vi "Test Internal Logic.vi"() -> ()   [LabVIEW 2020, in "Tamer.lvlib" / "Tamer.lvclass"]
uses:
  Tamer.lvclass
  Run Utilities/TypeDefs/Synchronize FPGA Cluster.ctl
  <vilib>/Utility/miscctls.llb/LVComboBoxStrsAndValuesArrayTypeDef.ctl
  Monkey Summary.ctl
  Run Utilities/TypeDefs/Monkey Status.ctl
  Link Chain GUI.ctl
  Reply.ctl
  Run Utilities/TypeDefs/Messages/Script Checker Message.ctl
  Run Utilities/TypeDefs/Script Checker Result.ctl
  af21684e-d11e-44f0-8b97-6f30b353b7a1.vi
  <vilib>/numeric/Random Number (Range) U64.vi
  d09a2809-11e4-490a-8cc9-e655e83ef35e.vi
  8c686b44-d516-4979-b4c0-187cf11809c2.vi
  <vilib>/numeric/sub_Random U32.vi
  <vilib>/Comparison/Less/Less Functor/Less Functor.lvclass
  Run Utilities/Run Utilities.lvlib
panel:
  in  "stop":bool
  in  "Tab Control":T1(tab)
  in  "Sync. Mask":T2[](array[typedef])=[{"Status"=FALSE, "FPGA Name"="Kasli 1"}, {"Status"=FALSE, "FPGA Name"="Kasli 1"}, {"Status"=TRUE, "FPGA Name"="Kasli 1"}]
  out "Synced Kaslis":string[](array[string])
  out "Number of Kaslis":i32
  out "Sync Process ID":string
  out "Processes":map{string, string[]}(c390)
  out "Synced Monkeys":string[](array[string])
  out "Number of Monkeys":i32
  out "key not found?":bool
  in  "Return Code recieved":string
  out "Return Code de-coded":T3(ring)
  in  "Status":string
  out "Status (enum)":T4=enum."Ongoing"
  in  "1D array in":string[](array[string])=["a00", "a01", "a10", "a11", "a20", "a21"]
  in  "columns":u32=1 min=1
  out "1D to 2D arry out":string[][](array[string])
  out "2D to 1D array out":string[](array[string])
  out "output array":T5
  in  "ADD":bool
  in  "REMOVE":bool
  in  "RESET":bool
  out "Value":string
  in  "Proc. Selector":string(combo)
  out "Size":i32
  out "added/deleted portion":cluster{"String":string, "Value":string}
  out "selected item":cluster{"String":string, "Value":string}
  in  "new Monkey":T6={"Color"=16777238, "Status"=enum."Init", "Continuous"=FALSE, "Scripts left"=0, "Scripts skipped"=0, "ETA"="", "Current Action"="", "Report from previous RUNs"="", "Monkey ID"="", "With DAQ?"=FALSE, "Linked?"=FALSE, "Paused"=FALSE}
  in  "Index":i32
  in  "SPAWN":bool
  in  "KILL":bool
  in  "KILL ALL":bool
  out "The Stage":T6[][](array[typedef])
  out "Monkey ID selected":string
  out "Guardians that have replied (unsorted)":T8[](array[typedef])
  out "Guardians that have replied (sorted)":T8[](array[typedef])
  out "Script Checker Results (unsorted)":T9[](array[typedef])
  out "Script Checker Results (sorted)":T9[](array[typedef])
  in  "Sync. Mask":T2[](array[typedef])=[{"Status"=FALSE, "FPGA Name"="Kasli 1"}, {"Status"=FALSE, "FPGA Name"="Kasli 1"}, {"Status"=TRUE, "FPGA Name"="Kasli 1"}]
  out "Kaslis":map{string, string}(c390)
  out "Monkeys Status in":map{string, T4}(c390)
  out "Monkeys":map{string, string[]}(c390)
  out "Processes in":map{string, string[]}(c390)
  out "Monkeys Status out":map{string, T4}(c390)
  out "Processes out":map{string, string[]}(c390)
  out "Kaslis out":map{string, string}(c390)
  out "Monkeys out":map{string, string[]}(c390)
  out "Sync Process ID":string
  in  "Monkey ID":string
  out "Sync Mask out":T2[](array[typedef])
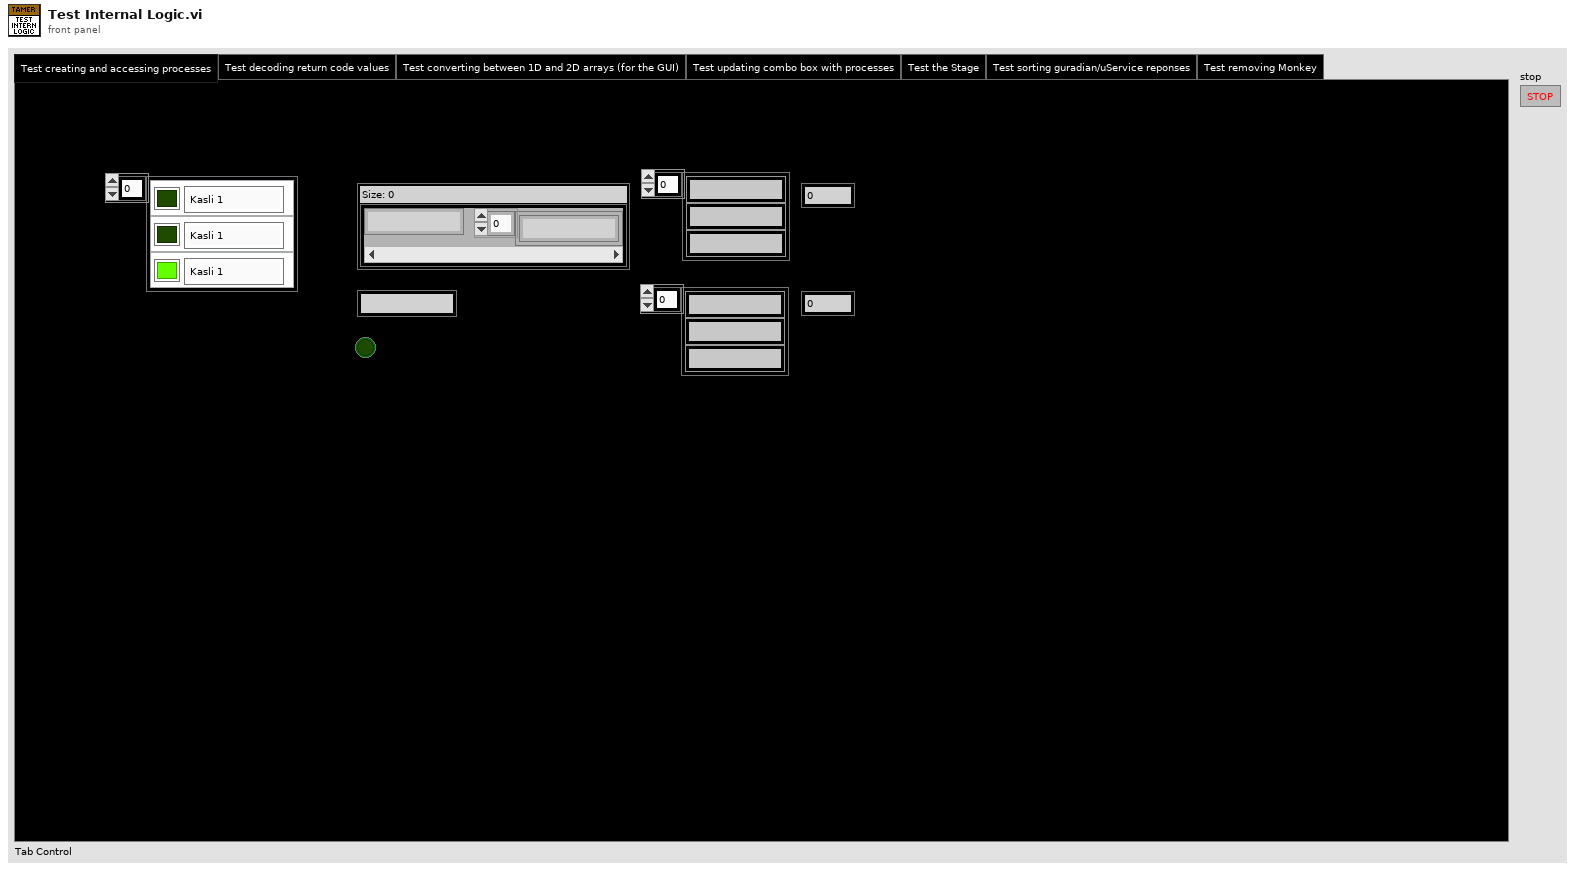
[diagram p1: front panel]
types:
  T1 = enum32{"Test creating and accessing processes", "Test decoding return code values", "Test converting between 1D and 2D arrays (for the GUI)", "Test updating combo box with processes", "Test the Stage", "Test sorting guradian/uService reponses", "Test removing Monkey"}
  T2 = typedef "Run Utilities.lvlib/Synchronize FPGA Cluster.ctl" = cluster{"Status":bool, "FPGA Name":string}
  T3 = enum16{"All Good", "Retry", "Skip", "Skip All", "ABORT"}
  T4 = typedef "Run Utilities.lvlib/Monkey Status.ctl" = enum16{"Init", "Paused", "Ongoing", "Stopped", "Finished (no errors)", "Finished (with errors)"}
  T5 = typedef "LVComboBoxStrsAndValuesArrayTypeDef.ctl" = cluster{"String":string, "Value":string}[]
  T6 = typedef "Tamer.lvlib/Tamer.lvclass/Monkey Summary.ctl" = cluster{"Color":u32, "Status":T4, "Continuous":bool, "Scripts left":u32, "Scripts skipped":u32, "ETA":string, "Current Action":string, "Report from previous RUNs":string, "Monkey ID":string, "With DAQ?":bool, "Linked?":T7, "Paused":bool}
  T7 = typedef "Tamer.lvlib/Tamer.lvclass/Link Chain GUI.ctl" = bool
  T8 = typedef "Tamer.lvlib/Tamer.lvclass/Reply.ctl" = cluster{"ID":string, "Status":bool, "GUID":string}
  T9 = typedef "Run Utilities.lvlib/Script Checker Message.ctl" = cluster{"Monkey ID":string, "Script Checker Result":T10}
  T10 = typedef "Run Utilities.lvlib/Script Checker Result.ctl" = enum16{"Passed", "Failed", "Empty"}
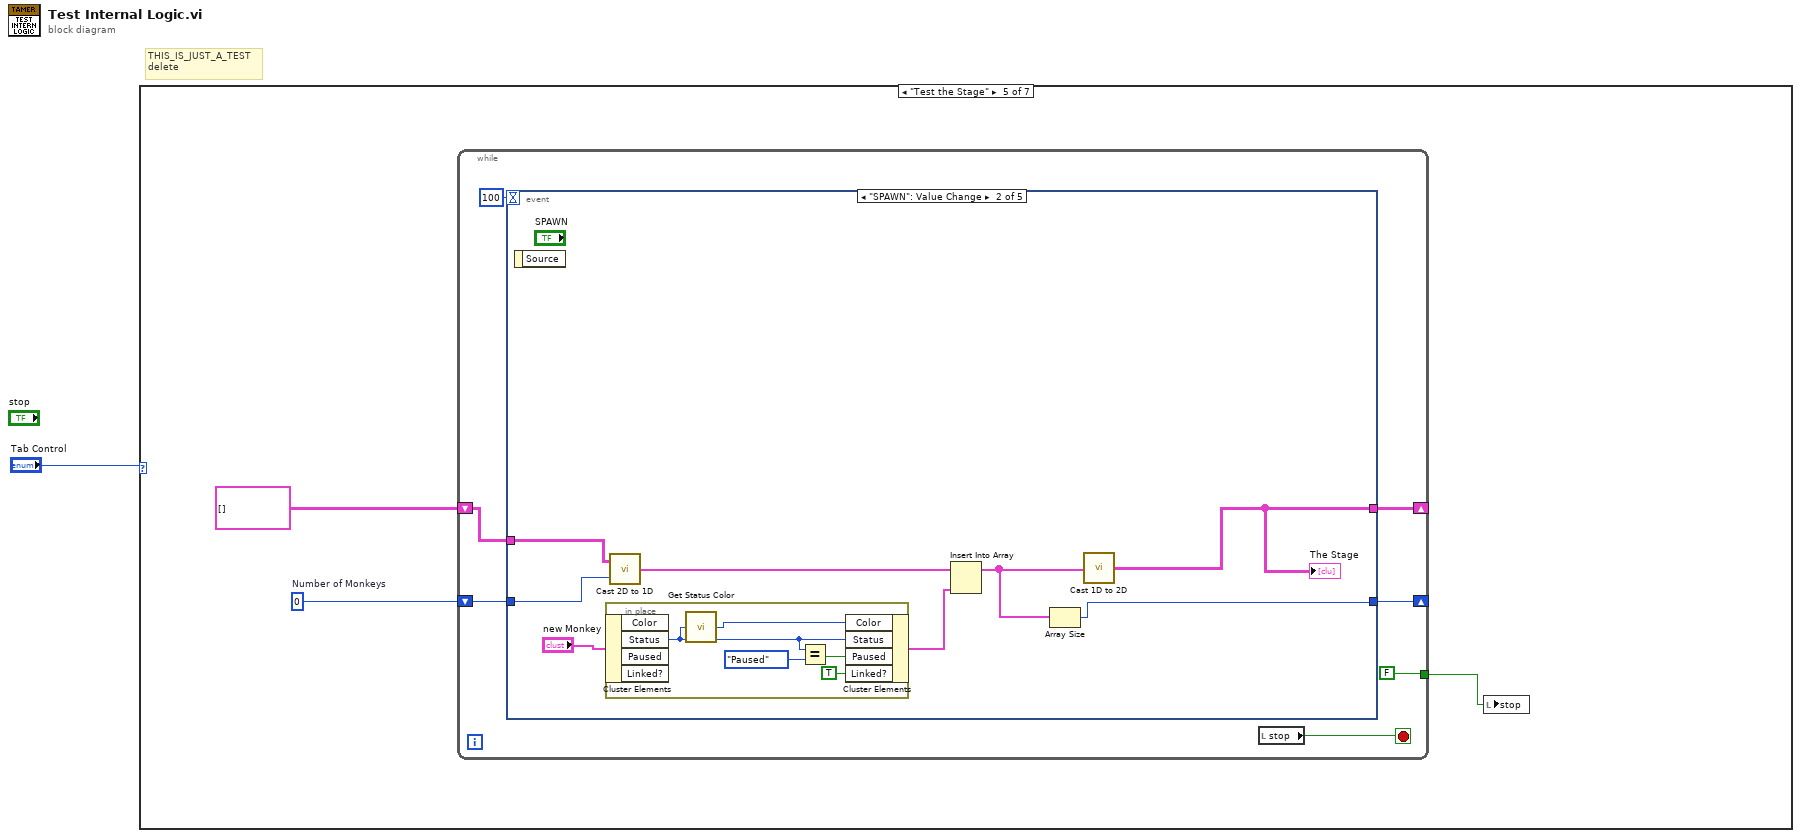
[diagram p0: block diagram]
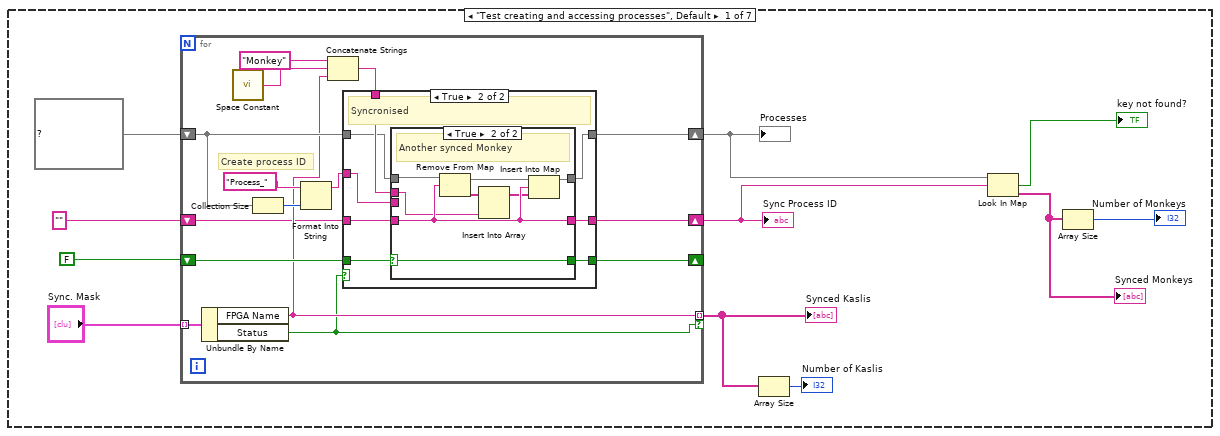
[diagram p2: hidden frame]
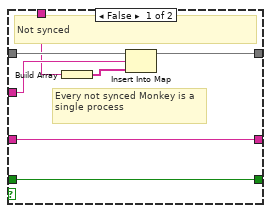
[diagram p3: hidden frame]
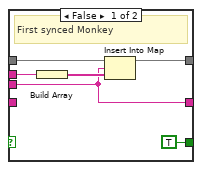
[diagram p4: hidden frame]
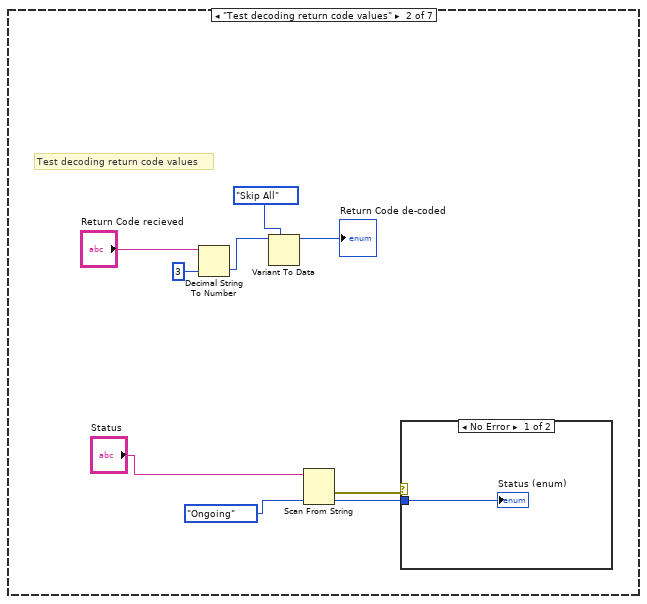
[diagram p5: hidden frame]
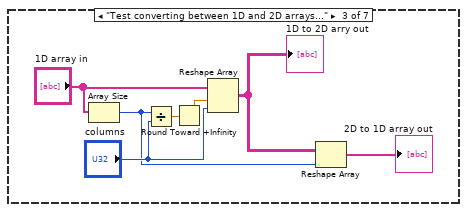
[diagram p7: hidden frame]
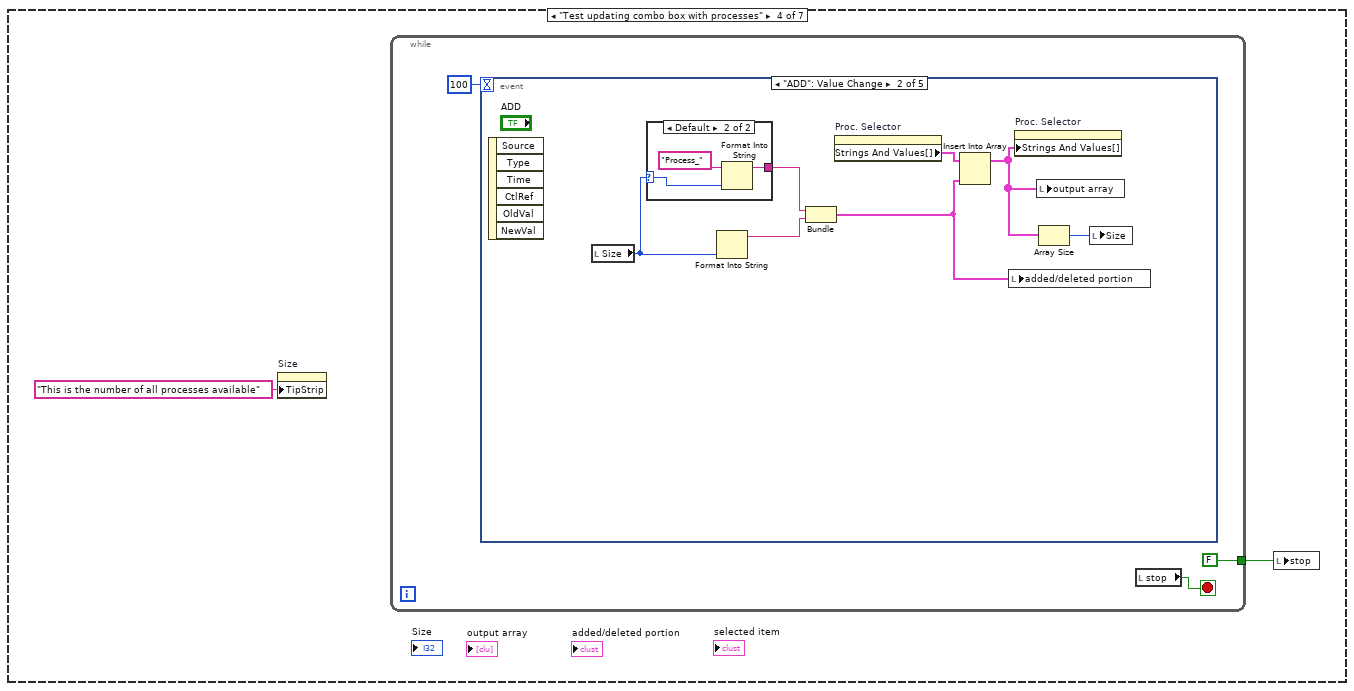
[diagram p8: hidden frame]
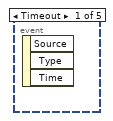
[diagram p9: hidden frame]
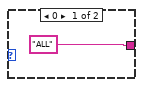
[diagram p10: hidden frame]
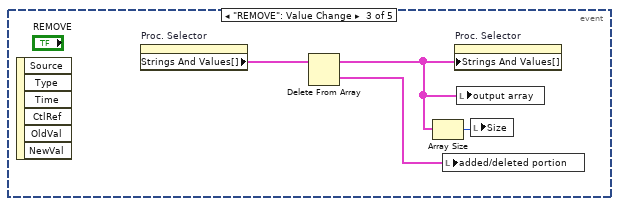
[diagram p11: hidden frame]
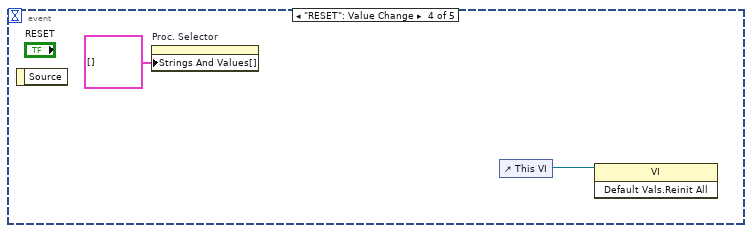
[diagram p12: hidden frame]
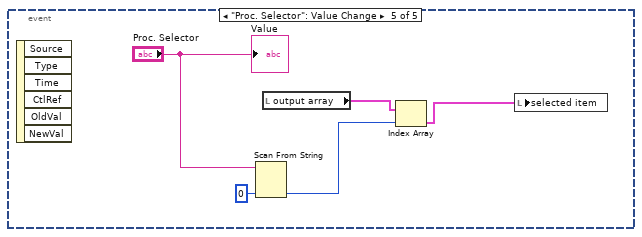
[diagram p13: hidden frame]
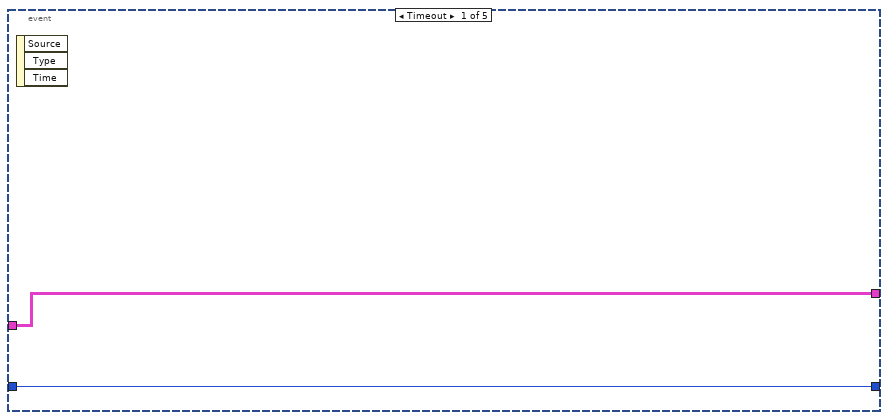
[diagram p14: hidden frame]
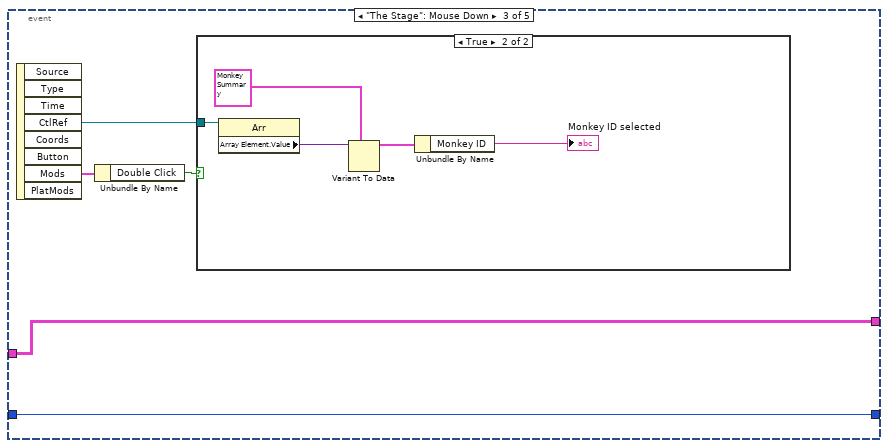
[diagram p15: hidden frame]
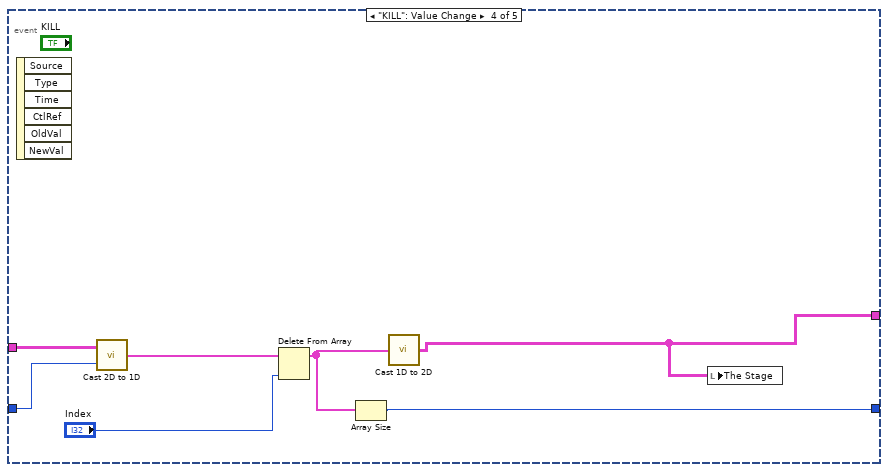
[diagram p17: hidden frame]
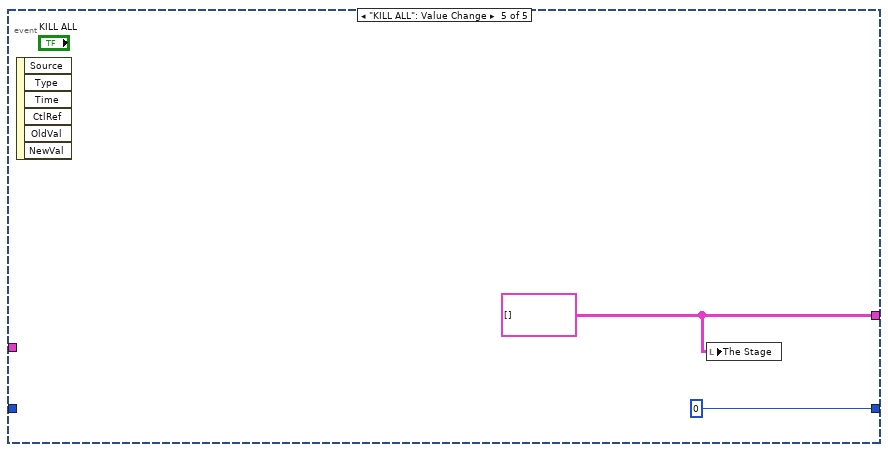
[diagram p18: hidden frame]
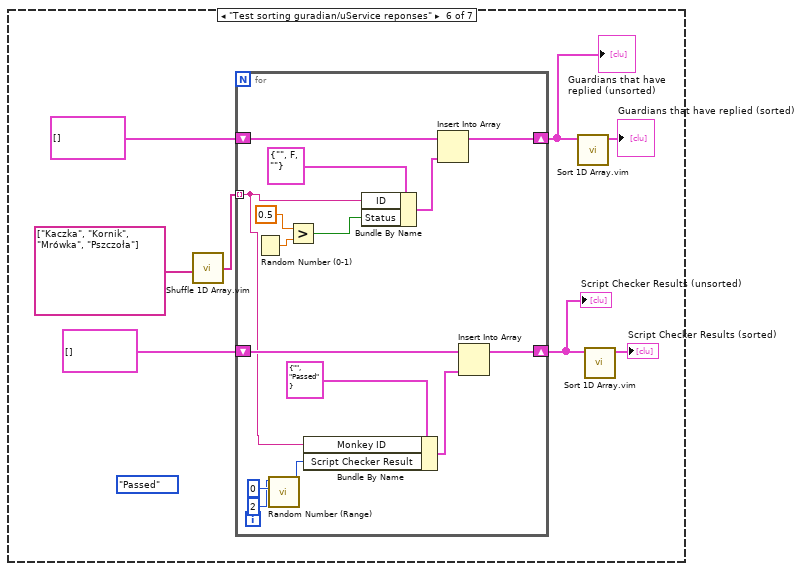
[diagram p19: hidden frame]
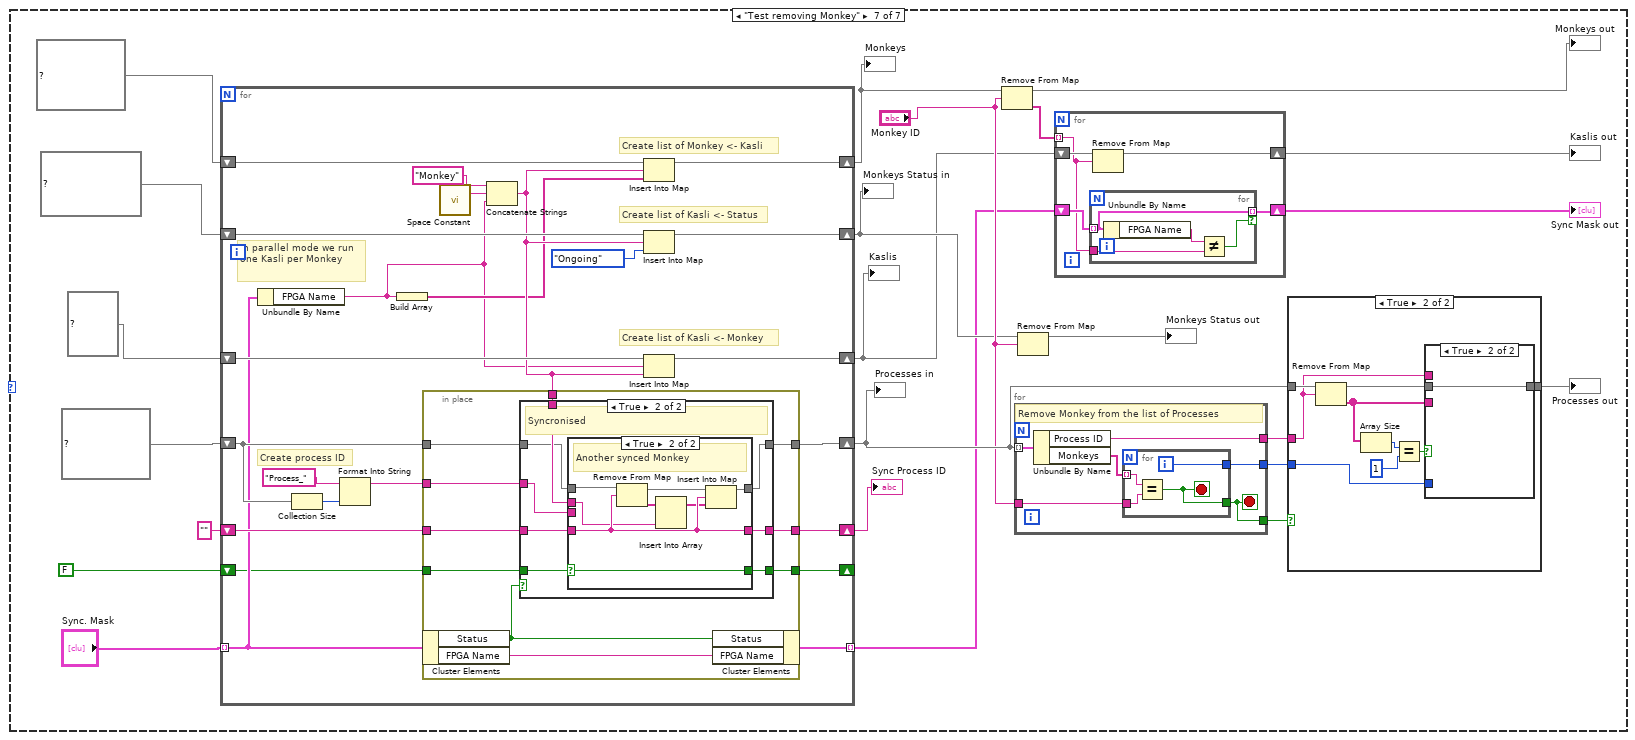
[diagram p20: hidden frame]
diagram:
  # "THIS_IS_JUST_A_TEST\ndelete"
  n1 = case shown="\"Test the Stage\"" "Tab Control" {
    frame "Test creating and accessing processes", Default {
      n2 = for {
        tunnel: "Sync. Mask" -> [w27] mode=indexing
        tunnel: [w17] -> w3 mode=indexing if=w13
        shift-right: [w26] -> w8
        shift-left: map{string, string[]} {} ("Processes") -> [w23]
        shift-right: [w21] -> _
        shift-left: FALSE ("Sync. Process added") -> [w22]
        shift-right: [w15] -> w9
        shift-left: "" -> [w14]
        # "Create process ID"
        n3 = Unbundle By Name(w27) -> ("FPGA Name"=w17:string, "Status"=w13:bool)
        n4 = call <vilib>:"Space Constant.vi"() -> ("String"=w18:string)
        n5 = Collection Size(1:w23) -> (0:w25:i32)
        n6 = Format Into String(initial string="Process_", w25) -> (resulting string=w20:string)  [unwired: 2 in, 1 out]
        n7 = Concatenate Strings("Monkey" ("string"), w18, w17) -> (w16:string)
        n8 = case shown="True" w13 {
          tunnel: w20 -> [w32 w38]
          tunnel: w23 -> [w34 w39]
          tunnel: [w33 w37] -> w26
          tunnel: w16 -> [w30 w41]
          tunnel: w22 -> [w29 w42]
          tunnel: [w29 w40] -> w21
          tunnel: [w28 w36] -> w15
          tunnel: w14 -> [w28 w35]
          frame False {
            # "Every not synced Monkey is a single process"
            # "Not synced"
            n9 = Build Array(w30) -> (w31:string[])
            n10 = Insert Into Map(map in=w34, key=w32, value=w31) -> (map out=w33:map{string, string[]})  [unwired: 2 out]
          }
          frame True {
            # "Syncronised"
            n11 = case shown="True" w42 {
              selector: w42 -> [_ w56]
              tunnel: [w46 w54] -> w37
              tunnel: w39 -> [w47 w55]
              tunnel: w41 -> [w45 w50]
              tunnel: [TRUE w56] -> w40
              tunnel: w38 -> [w43 _]
              tunnel: [w43 w52] -> w36
              tunnel: w35 -> [_ w52]
              frame False {
                # "First synced Monkey"
                n12 = Build Array(w45) -> (w44:string[])
                n13 = Insert Into Map(map in=w47, key=w43, value=w44) -> (map out=w46:map{string, string[]})  [unwired: 2 out]
              }
              frame True {
                # "Another synced Monkey"
                n14 = Remove From Map(10:w52, 11:w55) -> (1:w51:string[], 3:w53:map{string, string[]})  [unwired: 1 out]
                n15 = Insert Into Array(array=w51, new element=w50) -> (w49:string[])  [unwired: 1 in]
                n16 = Insert Into Map(map in=w53, key=w52, value=w49) -> (map out=w54:map{string, string[]})  [unwired: 2 out]
              }
            }
          }
        }
      }
      "Synced Kaslis" <- w3
      "Sync Process ID" <- w9
      "Processes" <- w8
      n17 = Array Size(array=w3) -> (size(s)=→"Number of Kaslis":i32)
      n18 = Look In Map(map=w8, key=w9) -> (key not found?=→"key not found?":bool, value=w10:string[])  [unwired: 1 in]
      "Synced Monkeys" <- w10
      n19 = Array Size(array=w10) -> (size(s)=→"Number of Monkeys":i32)
    }
    frame "Test decoding return code values" {
      # "Test decoding return code values"
      n20 = Decimal String To Number(string="Return Code recieved", default (0L)=3) -> (number=w65:i32)  [unwired: 1 in, 1 out]
      n21 = Variant To Data(type=T3."Skip All" ("Return Code"), Variant=w65) -> (data=→"Return Code de-coded":T3)  [unwired: 1 in, 1 out]
      n22 = Scan From String(input string="Status", default 1=Monkey_Status."Ongoing" ("Monkey Status")) -> (error out=w57:errorcluster, output 1=w58:T4)  [unwired: 3 in, 2 out]
      n23 = case shown="No Error" w57 {
        tunnel: w58 -> [w66 _]
        frame No Error {
          "Status (enum)" <- w66
        }
        frame Error {
        }
      }
    }
    frame "Test converting between 1D and 2D arrays (for the GUI)" {
      n24 = Array Size(array="1D array in") -> (size(s)=w69:i32)
      n25 = Divide(x=w69, y="columns") -> (x/y=w68:dbl)
      n26 = Round Toward +Infinity(x=w68) -> (ceil(x): smallest int >= x=w67:dbl)
      n27 = Reshape Array("1D array in", w67, "columns") -> (w71:string[][])
      "1D to 2D arry out" <- w71
      n28 = Reshape Array(w71, w69) -> (→"2D to 1D array out":string[])
    }
    frame "Test updating combo box with processes" {
      n29 = property on="Size" class="DigNum (strict)"("TipStrip"="This is the number of all processes available" ("Tip Strip")) -> ()  [unwired: 2 in, 2 out]
      n30 = while {
        tunnel: [FALSE] -> w75
        stop <- w77 stop-if-true
        n31 = event shown="[1] \"ADD\": Value Change" {
          selector: _ -> [_ _ _ _ _]
          dyn-events: _ -> [_ _ _ _ _]
          timeout: 100 -> [_ _ _ _ _]
          event Timeout {
            n32 = event-data() -> ()  [unwired: 1 in, 3 out]
          }
          event "ADD": Value Change {
            n33 = event-data() -> ()  [unwired: 1 in, 6 out]
            n34 = local read "Size"() -> (w82:i32)
            n35 = case shown="Default" w82 {
              selector: w82 -> [_ w88]
              tunnel: ["ALL" w87] -> w84
              frame 0 {
              }
              frame Default {
                n36 = Format Into String(initial string="Process_" ("string"), w88) -> (resulting string=w87:string)  [unwired: 2 in, 1 out]
              }
            }
            n37 = Format Into String(w82) -> (resulting string=w83:string)  [unwired: 3 in, 1 out]
            n38 = Bundle(w84, w83) -> (w79:cluster{string, string})  [unwired: 1 in]
            n39 = property on="Proc. Selector" class="CmbBox"() -> ("Strings And Values[]"=w85:T5)  [unwired: 2 in, 2 out]
            n40 = Insert Into Array(array=w85, new element=w79) -> (w80:T5)  [unwired: 1 in]
            n41 = local write "added/deleted portion"(w79) -> ()
            n42 = property on="Proc. Selector" class="CmbBox"("Strings And Values[]"=w80) -> ()  [unwired: 2 in, 2 out]
            n43 = local write "output array"(w80) -> ()
            n44 = Array Size(array=w80) -> (size(s)=w81:i32)
            n45 = local write "Size"(w81) -> ()
          }
          event "REMOVE": Value Change {
            n46 = event-data() -> ()  [unwired: 1 in, 6 out]
            n47 = property on="Proc. Selector" class="CmbBox"() -> ("Strings And Values[]"=w93:T5)  [unwired: 2 in, 2 out]
            n48 = Delete From Array(array=w93) -> (deleted portion=w92:cluster{"String":string, "Value":string}, array with subset deleted=w90:T5)  [unwired: 2 in]
            n49 = Array Size(array=w90) -> (size(s)=w91:i32)
            n50 = local write "added/deleted portion"(w92) -> ()
            n51 = property on="Proc. Selector" class="CmbBox"("Strings And Values[]"=w90) -> ()  [unwired: 2 in, 2 out]
            n52 = local write "output array"(w90) -> ()
            n53 = local write "Size"(w91) -> ()
          }
          event "RESET": Value Change {
            n54 = event-data() -> ()  [unwired: 1 in, 1 out]
            n55 = property on="Proc. Selector" class="CmbBox"("Strings And Values[]"=T5 [] ("Strings And Values []")) -> ()  [unwired: 2 in, 2 out]
            n56 = control-ref of="This VI"() -> (w95:refnum<vi>)
            n57 = invoke class="VI" method="Default Vals.Reinit All"(reference=w95) -> ()  [unwired: 2 in, 3 out]
          }
          event "Proc. Selector": Value Change {
            n58 = event-data() -> ()  [unwired: 1 in, 6 out]
            n59 = Scan From String(input string="Proc. Selector", default 1=0) -> (output 1=w96:i32)  [unwired: 3 in, 3 out]
            n60 = local read "output array"() -> (w100:T5)
            n61 = Index Array(array=w100, index=w96) -> (element=w99:cluster{"String":string, "Value":string})
            n62 = local write "selected item"(w99) -> ()
            "Value" <- "Proc. Selector"
          }
        }
        n63 = local read "stop"() -> (w77:bool)
      }
      n64 = local write "stop"(w75) -> ()
    }
    frame "Test the Stage" {
      w102 = 0  # Number of Monkeys
      n65 = while {
        shift-right: [w108] -> _
        shift-left: w102 -> [w109]
        shift-right: [w105] -> _
        shift-left: T6[][] [] ("The Cage") -> [w104]
        tunnel: [FALSE] -> w103
        stop <- w107 stop-if-true
        n66 = event shown="[1] \"SPAWN\": Value Change" {
          selector: _ -> [_ _ _ _ _]
          dyn-events: _ -> [_ _ _ _ _]
          timeout: 100 -> [_ _ _ _ _]
          tunnel: w109 -> [w112 w115 w128 w137 _]
          tunnel: [w111 w119 w129 w141 w143] -> w105
          tunnel: [w112 w117 w128 w139 0 ("Number of Monkeys")] -> w108
          tunnel: w104 -> [w111 w116 w129 w138 _]
          event Timeout {
            n67 = event-data() -> ()  [unwired: 1 in, 3 out]
          }
          event "SPAWN": Value Change {
            n68 = event-data() -> ()  [unwired: 1 in, 1 out]
            n69 = in-place {
              n70 = in-place-cluster #1("new Monkey") -> ("Status"=w124:T4)  [unwired: 3 out]
              n71 = call "Get Status Color.vi"("Monkey Status"=w124) -> ("Color"=w125:u32)
              n72 = Equal?(x=w124, y=Monkey_Status."Paused") -> (x = y?=w122:bool)
              n73 = in-place-cluster #1("Color"=w125, "Status"=w124, "Paused"=w122, "Linked?"=T7 TRUE) -> (w120:T6)
            }
            n74 = call "Cast 2D to 1D.vi"("1D size"=w115, "2D Synchronous Monkeys"=w116) -> ("1D Synchronous Monkeys"=w114:T6[])
            n75 = Insert Into Array(array=w114, new element=w120) -> (w118:T6[])  [unwired: 1 in]
            n76 = Array Size(array=w118) -> (size(s)=w117:i32)
            n77 = call "Cast 1D to 2D.vi"("1D Monkeys"=w118) -> ("2D Monkeys"=w119:T6[][])
            "The Stage" <- w119
          }
          event "The Stage": Mouse Down {
            n78 = event-data() -> ("CtlRef"=w130:refnum<vi>, "Mods"=w127:cluster{"Double Click":bool, "Menu Key":bool})  [unwired: 1 in, 6 out]
            n79 = Unbundle By Name(w127) -> ("Double Click"=w126:bool)
            n80 = case shown="True" w126 {
              tunnel: w130 -> [_ w135]
              frame False {
              }
              frame True {
                n81 = property class="Arr"(reference=w135) -> ("Array Element.Value"=w134:variant)  [unwired: 1 in, 2 out]
                n82 = Variant To Data(type=T6 {"Color"=16777238, "Status"=enum."Init", "Continuous"=FALSE, "Scripts left"=0, "Scripts skipped"=0, "ETA"="", "Current Action"="", "Report from previous RUNs"="", "Monkey ID"="", "With DAQ?"=FALSE, "Linked?"=FALSE, "Paused"=FALSE} ("Monkey Summary"), Variant=w134) -> (data=w133:T6)  [unwired: 1 in, 1 out]
                n83 = Unbundle By Name(w133) -> ("Monkey ID"=→"Monkey ID selected":string)
              }
            }
          }
          event "KILL": Value Change {
            n84 = event-data() -> ()  [unwired: 1 in, 6 out]
            n85 = call "Cast 2D to 1D.vi"("1D size"=w137, "2D Synchronous Monkeys"=w138) -> ("1D Synchronous Monkeys"=w136:T6[])
            n86 = Delete From Array(array=w136, index="Index") -> (array with subset deleted=w140:T6[])  [unwired: 1 in, 1 out]
            n87 = Array Size(array=w140) -> (size(s)=w139:i32)
            n88 = call "Cast 1D to 2D.vi"("1D Monkeys"=w140) -> ("2D Monkeys"=w141:T6[][])
            n89 = local write "The Stage"(w141) -> ()
          }
          event "KILL ALL": Value Change {
            w143 = T6[][] [] ("The Cage")
            n90 = event-data() -> ()  [unwired: 1 in, 6 out]
            n91 = local write "The Stage"(w143) -> ()
          }
        }
        n92 = local read "stop"() -> (w107:bool)
      }
      n93 = local write "stop"(w103) -> ()
    }
    frame "Test sorting guradian/uService reponses" {
      (unwired) Script_Checker_Result."Passed" ("Script Checker Result")
      n94 = call "Shuffle 1D Array.vim"("array"=string[] ["Kaczka", "Kornik", "Mrówka", "Pszczoła"]) -> ("shuffled array"=w151:string[])  [unwired: 4 in]
      n95 = for {
        shift-right: [w166] -> w149
        shift-left: T8[] [] ("Guardians that have replied") -> [w167]
        tunnel: w151 -> [w157] mode=indexing
        shift-right: [w159] -> w145
        shift-left: T9[] [] -> [w160]
        n96 = Random Number (0-1)() -> (number: 0 to 1=w163:dbl)
        n97 = call-poly <vilib>:"Random Number (Range).vi"("lower bound (0)"=u64 0, "upper bound (100)"=u64 2) -> ("number"=w154:u64)  [unwired: 9 in]
        n98 = Greater?(x=0.5, y=w163) -> (0:w161:bool)
        n99 = Bundle By Name(cluster=T9 {"Monkey ID"="", "Script Checker Result"=enum."Passed"} ("Message"), "Monkey ID"=w157, "Script Checker Result"=w154) -> (w153:T9)
        n100 = Bundle By Name(cluster=T8 {"ID"="", "Status"=FALSE, "GUID"=""} ("new element/subarray"), "ID"=w157, "Status"=w161) -> (w164:T8)
        n101 = Insert Into Array(array=w167, new element=w164) -> (w166:T8[])  [unwired: 1 in]
        n102 = Insert Into Array(array=w160, new element=w153) -> (w159:T9[])  [unwired: 1 in]
      }
      "Guardians that have replied (unsorted)" <- w149
      "Script Checker Results (unsorted)" <- w145
      n103 = call "Sort 1D Array.vim"("unsorted array"=w149) -> ("sorted array"=→"Guardians that have replied (sorted)":T8[])  [unwired: 10 in]
      n104 = call "Sort 1D Array.vim"("unsorted array"=w145) -> ("sorted array"=→"Script Checker Results (sorted)":T9[])  [unwired: 10 in]
    }
    frame "Test removing Monkey" {
      n105 = for {
        shift-right: [w248] -> w182
        shift-left: map{string, string[]} {} ("Monkeys") -> [w249]
        shift-right: [w246] -> w172
        shift-left: map{string, string} {} ("Kaslis") -> [w247]
        shift-right: [w244] -> w175
        shift-left: map{string, T4} {} ("Monkeys Status") -> [w245]
        tunnel: "Sync. Mask" -> [w234] mode=indexing
        tunnel: [w243] -> w169 mode=indexing
        shift-right: [w242] -> w180
        shift-left: map{string, string[]} {} ("Processes") -> [w239]
        shift-right: [w241] -> _
        shift-left: FALSE ("Sync. Process added") -> [w233]
        shift-right: [w235] -> w183
        shift-left: "" -> [w237]
        # "Create list of Kasli <- Monkey"
        # "Create list of Kasli <- Status"
        # "Create list of Monkey <- Kasli"
        # "Create process ID"
        # "In parallel mode we run one Kasli per Monkey"
        n106 = Unbundle By Name(w234) -> ("FPGA Name"=w227:string)
        n107 = Collection Size(1:w239) -> (0:w240:i32)
        n108 = Format Into String(initial string="Process_", w240) -> (resulting string=w236:string)  [unwired: 2 in, 1 out]
        n109 = Build Array(w227) -> (w228:string[])
        n110 = call <vilib>:"Space Constant.vi"() -> ("String"=w231:string)
        n111 = Concatenate Strings("Monkey" ("string"), w231, w227) -> (w229:string)
        n112 = in-place {
          in-place-border: [w256] -> w242
          in-place-border: w239 -> [w257]
          in-place-border: w233 -> [w253]
          in-place-border: [w252] -> w241
          in-place-border: w236 -> [w258]
          in-place-border: w229 -> [w255]
          in-place-border: w237 -> [w254]
          in-place-border: [w251] -> w235
          n113 = in-place-cluster #2(w234) -> ("Status"=w250:bool, "FPGA Name"=w259:string)
          n114 = case shown="True" w250 {
            tunnel: w258 -> [w264 w270]
            tunnel: w257 -> [w266 w271]
            tunnel: [w265 w269] -> w256
            tunnel: w255 -> [w262 w273]
            tunnel: w254 -> [w261 w267]
            tunnel: w253 -> [w260 w274]
            tunnel: [w260 w272] -> w252
            tunnel: [w261 w268] -> w251
            frame False {
              # "Every not synced Monkey is a single process"
              # "Not synced"
              n115 = Build Array(w262) -> (w263:string[])
              n116 = Insert Into Map(map in=w266, key=w264, value=w263) -> (map out=w265:map{string, string[]})  [unwired: 2 out]
            }
            frame True {
              # "Syncronised"
              n117 = case shown="True" w274 {
                selector: w274 -> [_ w288]
                tunnel: [w278 w286] -> w269
                tunnel: w271 -> [w279 w287]
                tunnel: w273 -> [w277 w282]
                tunnel: [TRUE w288] -> w272
                tunnel: w270 -> [w275 _]
                tunnel: [w275 w284] -> w268
                tunnel: w267 -> [_ w284]
                frame False {
                  # "First synced Monkey"
                  n118 = Build Array(w277) -> (w276:string[])
                  n119 = Insert Into Map(map in=w279, key=w275, value=w276) -> (map out=w278:map{string, string[]})  [unwired: 2 out]
                }
                frame True {
                  # "Another synced Monkey"
                  n120 = Remove From Map(10:w284, 11:w287) -> (1:w283:string[], 3:w285:map{string, string[]})  [unwired: 1 out]
                  n121 = Insert Into Array(array=w283, new element=w282) -> (w281:string[])  [unwired: 1 in]
                  n122 = Insert Into Map(map in=w285, key=w284, value=w281) -> (map out=w286:map{string, string[]})  [unwired: 2 out]
                }
              }
            }
          }
          n123 = in-place-cluster #2("Status"=w250, "FPGA Name"=w259) -> (w243:T2)
        }
        n124 = Insert Into Map(map in=w249, key=w229, value=w228) -> (map out=w248:map{string, string[]})  [unwired: 2 out]
        n125 = Insert Into Map(map in=w245, key=w229, value=Monkey_Status."Ongoing") -> (map out=w244:map{string, T4})  [unwired: 2 out]
        n126 = Insert Into Map(map in=w247, key=w227, value=w229) -> (map out=w246:map{string, string})  [unwired: 2 out]
      }
      "Kaslis" <- w172
      "Monkeys" <- w182
      "Monkeys Status in" <- w175
      "Processes in" <- w180
      "Sync Process ID" <- w183
      n127 = Remove From Map(10:"Monkey ID", 11:w182) -> (1:w173:string[], 3:→"Monkeys out":map{string, string[]})  [unwired: 1 out]
      n128 = for {
        tunnel: w180 -> [w222] mode=indexing
        tunnel: "Monkey ID" -> [w220]
        tunnel: [w219] -> w178
        tunnel: [w218] -> w179
        tunnel: [w217] -> w170
        stop <- w217 stop-if-true
        # "Remove Monkey from the list of Processes"
        n129 = Unbundle By Name(w222) -> ("Process ID"=w219:string, "Monkeys"=w221:string[])
        n130 = for {
          tunnel: w221 -> [w226] mode=indexing
          tunnel: w220 -> [w225]
          tunnel: [w224] -> w217
          tunnel: [w223] -> w218
          i -> [w223]
          stop <- w224 stop-if-true
          n131 = Equal?(x=w226, y=w225) -> (x = y?=w224:bool)
        }
      }
      n132 = Remove From Map(10:"Monkey ID", 11:w175) -> (3:→"Monkeys Status out":map{string, T4})  [unwired: 2 out]
      n133 = for {
        tunnel: w173 -> [w209] mode=indexing
        shift-right: [w211] -> w171
        shift-left: w172 -> [w212]
        shift-right: [w208] -> w168
        shift-left: w169 -> [w210]
        n134 = for {
          tunnel: w210 -> [w214] mode=indexing
          tunnel: w209 -> [w215]
          tunnel: [w214] -> w208 mode=indexing if=w213
          n135 = Unbundle By Name(w214) -> ("FPGA Name"=w216:string)
          n136 = Not Equal?(x=w216, y=w215) -> (x != y?=w213:bool)
        }
        n137 = Remove From Map(10:w209, 11:w212) -> (3:w211:map{string, string})  [unwired: 2 out]
      }
      "Kaslis out" <- w171
      "Sync Mask out" <- w168
      n138 = case shown="True" w170 {
        tunnel: w180 -> [w191 w200]
        tunnel: w179 -> [_ w194]
        tunnel: w178 -> [_ w193]
        tunnel: [w191 w192] -> w177
        frame False {
        }
        frame True {
          n139 = Remove From Map(10:w193, 11:w200) -> (1:w195:string[], 3:w196:map{string, string[]})  [unwired: 1 out]
          n140 = Array Size(array=w195) -> (size(s)=w199:i32)
          n141 = Equal?(x=w199, y=1) -> (x = y?=w197:bool)
          n142 = case shown="True" w197 {
            tunnel: w196 -> [w204 w207]
            tunnel: [w201 w207] -> w192
            tunnel: w195 -> [w206 _]
            tunnel: w194 -> [w205 _]
            tunnel: w193 -> [w203 _]
            frame False {
              n143 = Delete From Array(array=w206, index=w205) -> (array with subset deleted=w202:string[])  [unwired: 1 in, 1 out]
              n144 = Insert Into Map(map in=w204, key=w203, value=w202) -> (map out=w201:map{string, string[]})  [unwired: 2 out]
            }
            frame True {
            }
          }
        }
      }
      "Processes out" <- w177
    }
  }
